vi "XY Graph Get Selected Plots.vi"(8 "error in (no error)":errorcluster, 11 "XYGraph in":T1) -> (0 "error out":errorcluster, 1 "Selected Plots":i32[](array[numeric]), 2 "Selected Plot Names":string[](array[string]), 3 "XYGraph out":T1, 5 "Graph Caption":string)   [LabVIEW 2019, in "XY Graph Add-Ons.lvlib"]
uses:
  XY Graph Add-Ons.lvlib
  XY Graph Refnum.ctl
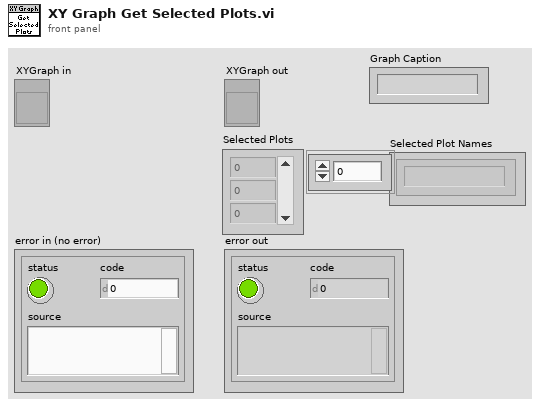
[diagram p1: front panel]
types:
  T1 = typedef "XY Graph Add-Ons.lvlib/XY Graph Refnum.ctl" = refnum<vi>
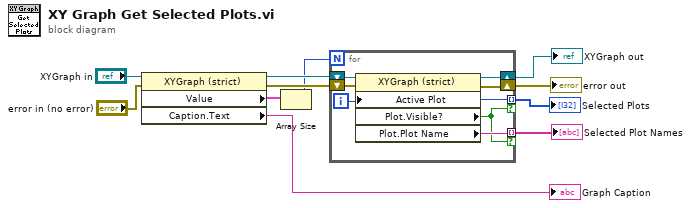
[diagram p0: block diagram]
diagram:
  n1 = property class="XYGraph (strict)"(reference="XYGraph in", error in="error in (no error)") -> (reference out=w8:T1, error out=w7:errorcluster, "Value"=w10:cluster{"X Array":dbl[], "Y Array":dbl[]}[], "Caption.Text"=→"Graph Caption":string)
  n2 = Array Size(array=w10) -> (size(s)=w3:i32)
  n3 = for {
    N: w3 -> [_]
    shift-right: [w17] -> w6
    shift-left: w8 -> [w18]
    tunnel: [w15] -> w4 mode=indexing if=w12
    shift-right: [w14] -> w5
    shift-left: w7 -> [w16]
    tunnel: [w13] -> w2 mode=indexing if=w12
    i -> [w15]
    n4 = property class="XYGraph (strict)"(reference=w18, error in=w16, "Active Plot"=w15) -> (reference out=w17:T1, error out=w14:errorcluster, "Plot.Visible?"=w12:bool, "Plot.Plot Name"=w13:string)
  }
  "XYGraph out" <- w6
  "error out" <- w5
  "Selected Plots" <- w4
  "Selected Plot Names" <- w2
